vi "Find VIPath From VIName (In Memory).vi"(10 "VI Name":string) -> (2 "VI Path":path)   [LabVIEW 2021, in "Bananas.lvlib"]
uses:
  Bananas.lvlib
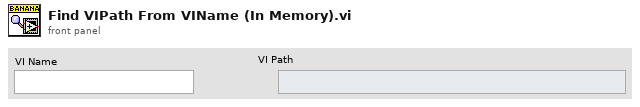
[diagram p1: front panel]
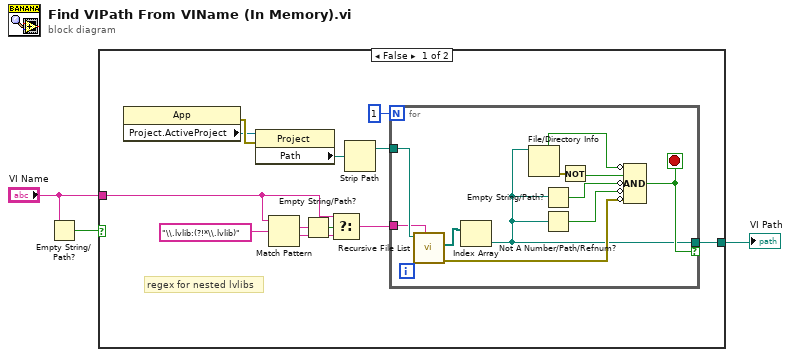
[diagram p0: block diagram]
diagram:
  n1 = Empty String/Path?(string/path="VI Name") -> (empty?=w1:bool)
  n2 = case shown="False" w1 {
    tunnel: [w15 _] -> w3
    tunnel: "VI Name" -> [w4 _]
    frame False {
      # "regex for nested lvlibs"
      n3 = property class="App"() -> (error out=w7:errorcluster, "Project.ActiveProject"=w5:refnum<vi>)  [unwired: 2 in, 1 out]
      n4 = property class="Project"(reference=w5, error in=w7) -> ("Path"=w6:path)  [unwired: 2 out]
      n5 = Match Pattern(string=w4, regular expression="\\.lvlib:(?!*\\.lvlib)") -> (match substring=w10:string, after substring=w8:string)  [unwired: 1 in, 2 out]
      n6 = Empty String/Path?(string/path=w10) -> (empty?=w9:bool)
      n7 = Select(t=w4, s=w9, f=w8) -> (s? t:f=w12:string)
      n8 = Strip Path(path=w6) -> (stripped path=w13:path)  [unwired: 1 out]
      n9 = for {
        N: 1 -> [_]
        tunnel: [w17] -> w15 if=w24
        tunnel: w12 -> [w22]
        tunnel: w13 -> [w23]
        stop <- w24 stop-if-true
        n10 = call <vilib>:"Recursive File List.vi"("pattern"=w22, "Folder Path"=w23) -> ("error out"=w21:errorcluster, "All Files in Dir"=w20:path[])  [unwired: 5 in, 3 out]
        n11 = Index Array(array=w20) -> (element=w17:path)  [unwired: 1 in]
        n12 = File/Directory Info(path=w17) -> (directory=w19:bool, error out=w16:errorcluster)  [unwired: 1 in, 5 out]
        n13 = Empty String/Path?(string/path=w17) -> (empty?=w26:bool)
        n14 = Not A Number/Path/Refnum?(number/path/refnum=w17) -> (NaN/Path/Refnum?=w25:bool)
        n15 = Not(x=w16) -> (.not. x?=w18:bool)
        n16 = Compound Arithmetic op=AND(invert w19, w18, invert w26, invert w25, invert w21) -> (w24:bool)
      }
    }
    frame True {
    }
  }
  "VI Path" <- w3
